vi "Apply ROIs.vi"(7 "Mode (Redraw All)":enum16{"Redraw All", "Draw Last"}(ring), 8 "error in (no error)":errorcluster, 9 "ROIs Info []":T1[](array[typedef]) {"Zoom" min=1.0 max=10.0 step=0.10000000149011612}) -> (0 "error out":errorcluster, 1 "Number of ROI":i32, 2 "Cycle time (us)":dbl, 3 "No ROI":bool)   [LabVIEW 2013]
uses:
  Typedefs/ROI spec.ctl
  Typedefs/ROI ID Enum.ctl
  Typedefs/ROI management FG states.ctl
  Typedefs/ROI management Input cluster.ctl
  Global Variables/General Globals.vi
  <resource>/objmgr/IMAQImage.rc
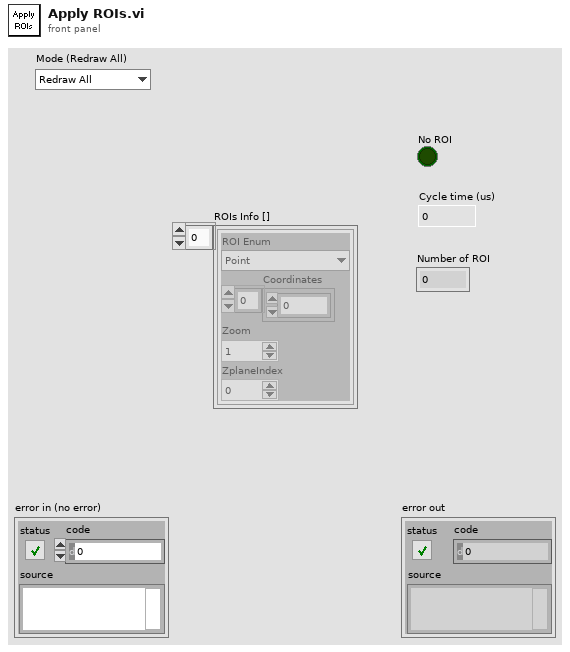
[diagram p1: front panel]
types:
  T1 = typedef "ROI spec.ctl" = cluster{"Coordinates":i32[], "Zoom":dbl, "ROI Enum":T2, "ZplaneIndex":i32}
  T2 = typedef "ROI ID Enum.ctl" = enum16{"Point", "MiniScan", "Comp. MiniScan", "Rectangle", "Comp. volume", "Arb. plane point"}
  T3 = typedef "ROI management FG states.ctl" = enum16{"Read", "Write", "Clear Last", "Clear All", "Update ROIs time", "Reload last ROI set", "Offset all ROI", "Offset visible ROI"}
  T4 = typedef "ROI parameters data type.ctl" = cluster{"ROI index":dbl, "ROI ID":dbl, "ROI Time (ns)":dbl, "Pixels in ROI":dbl, "X start":dbl, "Y start":dbl, "Z start":dbl, "X stop":dbl, "Y stop":dbl, "Z stop":dbl, "Angle (deg)":dbl, "Composite ID":dbl, "Number of lines":dbl, "Frame Size":dbl, "Zoom":dbl, "Laser Power (%)":dbl, "ROI group ID":dbl}
  T5 = typedef "ROI management Input cluster.ctl" = cluster{"ROI Type":T2, "XY Coordinates":i32[], "Motor Z Planes":dbl[], "ZPlane Index":i32, "Dwell time per POI or per pixel (us)":dbl, "Frame size":i32, "Zoom":dbl}
  T6 = typedef "IMAQ Image.ctl" = refnum<image>
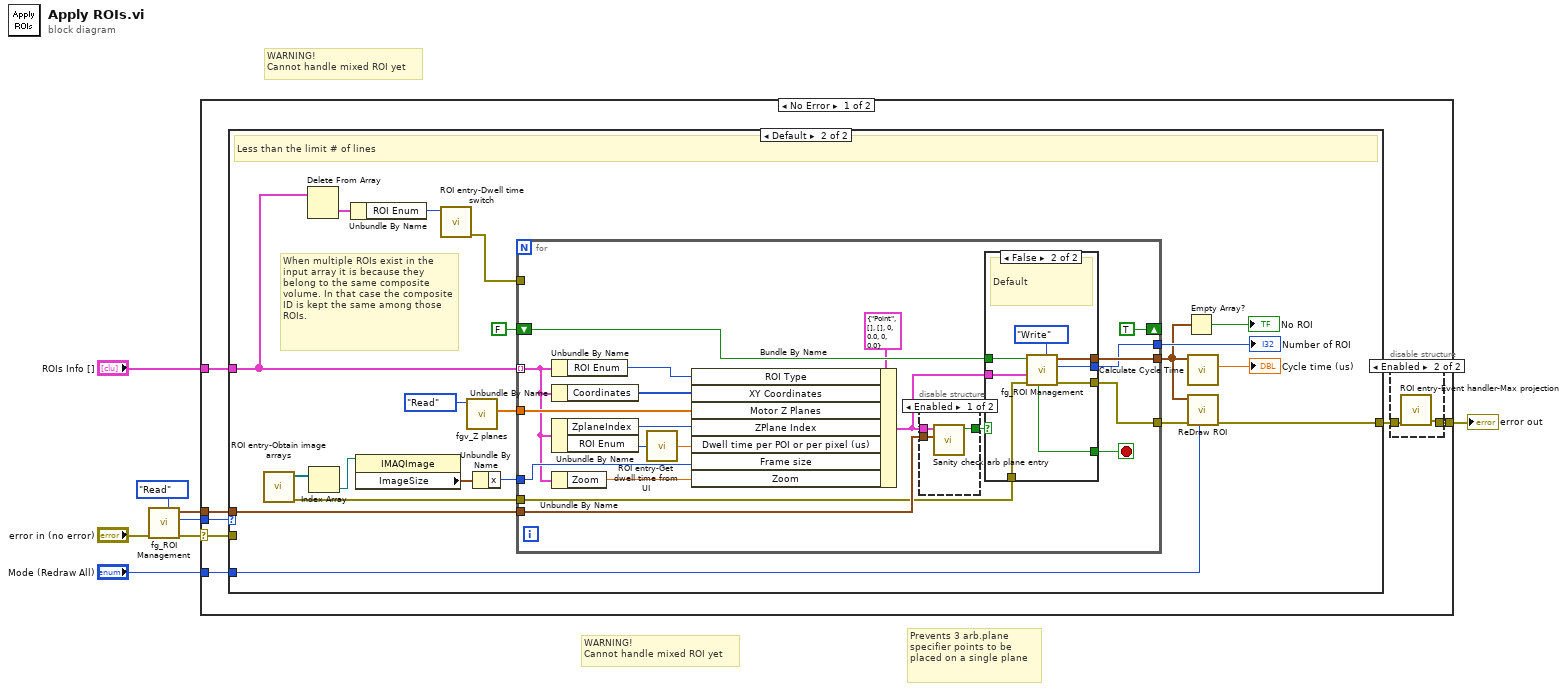
[diagram p0: block diagram]
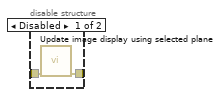
[diagram p2: hidden frame]
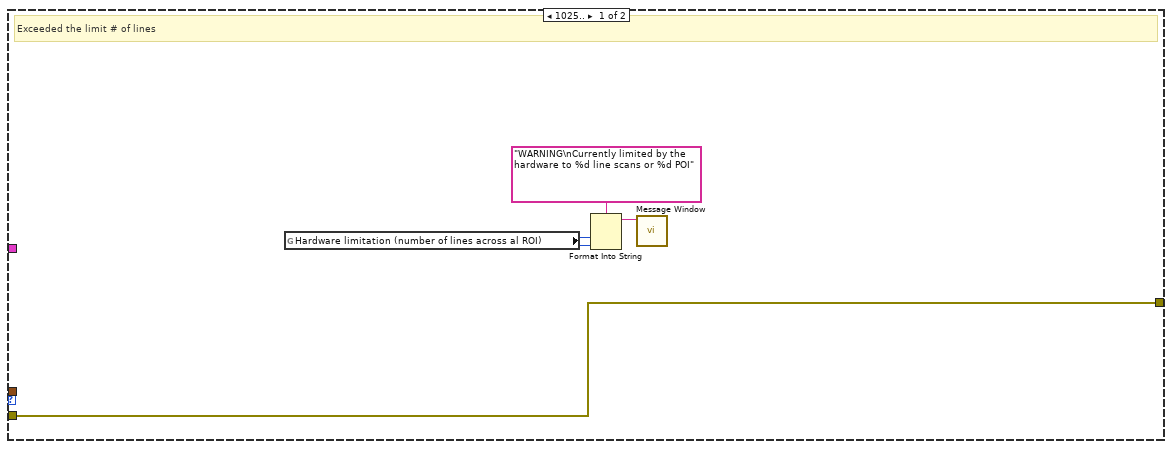
[diagram p3: hidden frame]
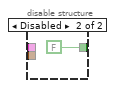
[diagram p4: hidden frame]
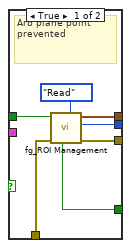
[diagram p5: hidden frame]
diagram:
  # "WARNING!\nCannot handle mixed ROI yet"
  # "WARNING!\nCannot handle mixed ROI yet"
  # "Prevents 3 arb.plane specifier points to be placed on a single plane"
  n1 = call "fg_ROI Management.vi"("Function"=ROI_management_FG_states."Read", "error in (no error)"="error in (no error)") -> ("error out"=w3:errorcluster, "Number of ROI"=w5:i32, "ROI Setup"=w4:T4[])  [unwired: 5 in, 2 out]
  n2 = case shown="No Error" w3 {
    selector: w3 -> [w12 w83]
    tunnel: w5 -> [w15 _]
    tunnel: w4 -> [w14 _]
    tunnel: [w10 w83] -> w2
    tunnel: "ROIs Info []" -> [w13 _]
    tunnel: "Mode (Redraw All)" -> [w9 _]
    frame No Error {
      n3 = case shown="Default" w15 {
        tunnel: w14 -> [_ w37]
        tunnel: w13 -> [_ w27]
        tunnel: [w23 w33] -> w11
        tunnel: w12 -> [w23 _]
        tunnel: w9 -> [_ w28]
        frame 1025.. {
          # "Exceeded the limit # of lines"
          n4 = global read "General Globals.vi" "Hardware limitation (number of lines across al ROI)"() -> (w20:i32)
          n5 = Format Into String(format string="WARNING\nCurrently limited by the hardware to %d line scans or %d POI" ("Message string"), w20, w20) -> (resulting string=w21:string)  [unwired: 2 in, 1 out]
          n6 = call "Message Window.vi"("Message string"=w21) -> ()  [unwired: 10 in, 1 out]
        }
        frame Default {
          # "When multiple ROIs exist in the input array it is because they belong to the same composite volume. In that case the composite ID is kept the same among those ROIs."
          # "Less than the limit # of lines"
          n7 = call "ROI entry-Obtain image arrays.vi"() -> ("error IO"=w32:errorcluster, "RedImageArray"=w36:T6[])  [unwired: 10 in]
          n8 = Delete From Array(array=w27) -> (deleted portion=w26:T1)  [unwired: 2 in, 1 out]
          n9 = Index Array(array=w36) -> (element=w41:T6)  [unwired: 1 in]
          n10 = Unbundle By Name(w26) -> ("ROI Enum"=w25:T2)
          n11 = property class="IMAQImage"(reference=w41) -> ("ImageSize"=w40:cluster{"x":i32, "y":i32})  [unwired: 1 in, 2 out]
          n12 = call "ROI entry-Dwell time switch.vi"("ROI Enum"=w25) -> ("error out"=w24:errorcluster)  [unwired: 10 in]
          n13 = call "fgv_Z planes.vi"("Function"=enum16{"Intialize", "Write", "Read", "Clear"}."Read") -> ("AOL Z Planes"=w34:dbl[])  [unwired: 8 in, 2 out]
          n14 = Unbundle By Name(w40) -> ("x"=w39:i32)
          n15 = for {
            tunnel: [w63] -> w30
            tunnel: w27 -> [w46] mode=indexing
            tunnel: w34 -> [w59]
            shift-right: [TRUE] -> _
            shift-left: FALSE -> [w62]
            tunnel: w39 -> [w58]
            tunnel: [w54] -> w38
            tunnel: w37 -> [w52]
            tunnel: w32 -> [w50]
            tunnel: [w49] -> w31
            tunnel: w24 -> [_]
            stop <- w55 stop-if-true
            n16 = Unbundle By Name(w46) -> ("ROI Enum"=w48:T2)
            n17 = Unbundle By Name(w46) -> ("Coordinates"=w57:i32[])
            n18 = Unbundle By Name(w46) -> ("ZplaneIndex"=w45:i32, "ROI Enum"=w44:T2)
            n19 = Unbundle By Name(w46) -> ("Zoom"=w56:dbl)
            n20 = call "ROI entry-Get dwell time from UI.vi"("ROI Enum"=w44) -> ("Dynamic dwell time(us)"=w47:dbl)
            n21 = Bundle By Name(cluster=T5 {"ROI Type"=enum."Point", "XY Coordinates"=[], "Motor Z Planes"=[], "ZPlane Index"=0, "Dwell time per POI or per pixel (us)"=0.0, "Frame size"=0, "Zoom"=0.0} ("ROI management Input cluster"), "ROI Type"=w48, "XY Coordinates"=w57, "Motor Z Planes"=w59, "ZPlane Index"=w45, "Dwell time per POI or per pixel (us)"=w47, "Frame size"=w58, "Zoom"=w56) -> (w53:T5)
            n22 = disable-structure shown="Enabled" {
              disable-tunnel: w53 -> [w66 _]
              disable-tunnel: w52 -> [w65 _]
              disable-tunnel: [w64 FALSE ("Prevent new POI")] -> w51
              frame Enabled {
                n23 = call "Sanity check arb plane entry.vi"("ROI Setup"=w65, "ROI management Input cluster"=w66) -> ("Prevent new POI"=w64:bool)  [unwired: 9 in]
              }
              frame Disabled {
              }
            }
            n24 = case shown="False" w51 {
              tunnel: [w74 w82] -> w63
              tunnel: w62 -> [w73 w81]
              tunnel: [w72 w80] -> w55
              tunnel: [w70 w78] -> w54
              tunnel: w53 -> [_ w77]
              tunnel: w50 -> [w69 w76]
              tunnel: [w68 w75] -> w49
              frame True {
                # "Arb plane point prevented"
                n25 = call "fg_ROI Management.vi"("Function"=ROI_management_FG_states."Read", "error in (no error)"=w69, "Reuse last composite ID"=w73) -> ("error out"=w68:errorcluster, "Number of ROI"=w70:i32, "ROI Setup"=w74:T4[], "Exceeded limit number of lines"=w72:bool)  [unwired: 4 in, 1 out]
              }
              frame False {
                # "Default"
                n26 = call "fg_ROI Management.vi"("Function"=ROI_management_FG_states."Write", "error in (no error)"=w76, "ROI management Input cluster"=w77, "Reuse last composite ID"=w81) -> ("error out"=w75:errorcluster, "Number of ROI"=w78:i32, "ROI Setup"=w82:T4[], "Exceeded limit number of lines"=w80:bool)  [unwired: 3 in, 1 out]
              }
            }
          }
          "Number of ROI" <- w38
          n27 = Empty Array?(array=w30) -> (empty?=→"No ROI":bool)
          n28 = call "Calculate Cycle Time.vi"("Coordinates"=w30) -> ("Cycle time (us)"=→"Cycle time (us)":dbl)  [unwired: 9 in, 1 out]
          n29 = call "ReDraw ROI.vi"("Mode (Redraw All)"=w28, "error in"=w31, "XYZ Coordinates"=w30) -> ("error out"=w33:errorcluster)  [unwired: 8 in]
        }
      }
      n30 = disable-structure shown="Enabled" {
        disable-tunnel: w11 -> [w17 w19]
        disable-tunnel: [w16 w18] -> w10
        frame Disabled {
          n31 = call "Update image display using selected plane.vi"("error in (no error)"=w17) -> ("error out"=w16:errorcluster)  [unwired: 10 in]
        }
        frame Enabled {
          n32 = call "ROI entry-Event handler-Max projection.vi"("error in (no error)"=w19) -> ("error out"=w18:errorcluster)  [unwired: 10 in]
        }
      }
    }
    frame Error {
    }
  }
  "error out" <- w2
